vi "Testing Mode.vi"(8 "Filepath":path=path "D:/My Project/2019-2020/Magnetic Mareli UM/MM_UM/Project Setup/data/program seq/Program_280A.bin", 9 "FeedBack Channel":string[](array[string])=["fgdgfvcbc", "vnfhgjkn", "21354682"]) -> ()   [LabVIEW 2015]
uses:
  Control Button/Exit.ctl
  Control Button/Start.ctl
  Control Button/Home call.ctl
  Test  enqueue/AutoTest seq.ctl
  Control Button/Stop.ctl
  Control Button/Emergency.ctl
  Test  enqueue/Auot Test selection.ctl
  Galobal variable_TI.vi
  Project Setup/Globle Variable/GR_Servo.vi
panel:
  out "XY Graph":cluster{"X":dbl, "Y":dbl}[](graph)
  in  "Emergency":T1
  in  "Stop":T2
  out "Digital Output":bool[](array[boolean])
  out "D-enqueue":T3
  in  "Home Call":bool
  out "DI":bool[](array[boolean])
  in  "Home":T4
  out "Error Message":string
  out "Current Date & Time":timestamp
  out "Cycle Time(Sec)":i32
  in  "Start":T5
  in  "Cycle Start Bit":bool
  in  "vi reference":refnum<vi>
  in  "Reset Ct.":bool
  out "error out":errorcluster
  in  "Tbl Refnum":refnum<vi>
  in  "Table Control":string[][](table)
  out "User Name":string
  in  "Image Display":bool
  in  "Exit":T6
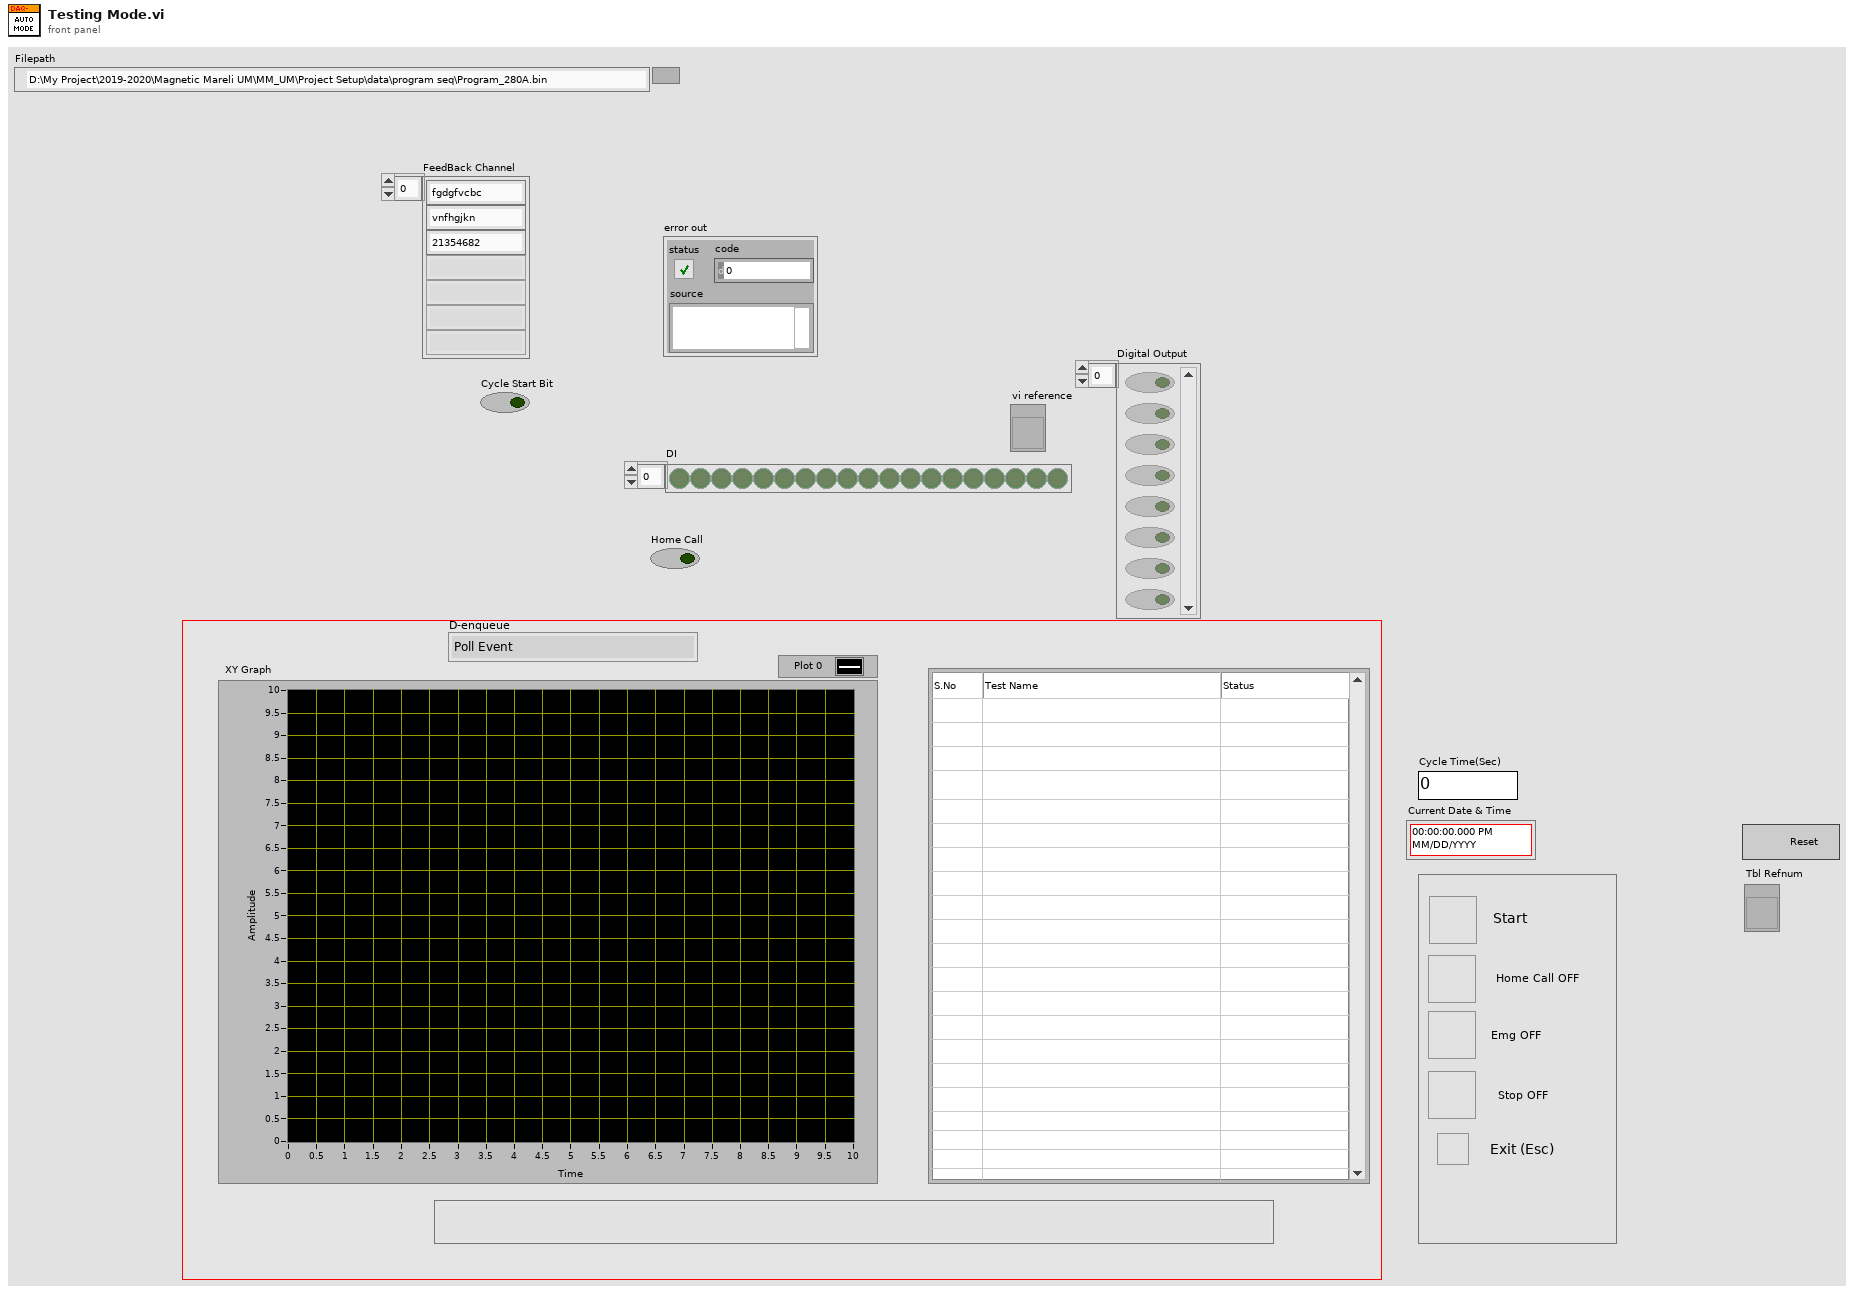
[diagram p1: front panel]
types:
  T1 = typedef "Emergency.ctl" = bool
  T2 = typedef "Stop.ctl" = bool
  T3 = typedef "AutoTest seq.ctl" = enum16{"Poll Event", "Initilization", "Cylender Home", "Read Barcode", "Slide Servo send Cammand", "Slide Servo Home Call", "LCD Press Servo send Cammand", "LCD Press. Servo Home Call", "Camera Co-ordinate_1", "Camera Co-ordinate_2", "Result Save", "Exit"}
  T4 = typedef "Home call.ctl" = bool
  T5 = typedef "Start.ctl" = bool
  T6 = typedef "Exit.ctl" = bool
  T7 = typedef "Auot Test selection.ctl" = enum16{"Init", "Enqueue ", "Enqueue N", "Enqueue in stack", "Enqueue in stack N", "Dequeue", "Dequeue N", "Flush", "Release Queue"}
  T8 = cluster{"Item Name":string, "Item Status":bool, "Steps":cluster{"Channel Type":string, "Channels":string, "Wait/Poll (ms)":u32, "Parameter":u8, "STM-Speed":i32, "STM-Degree":u32, "Direction":u8}[]}[]
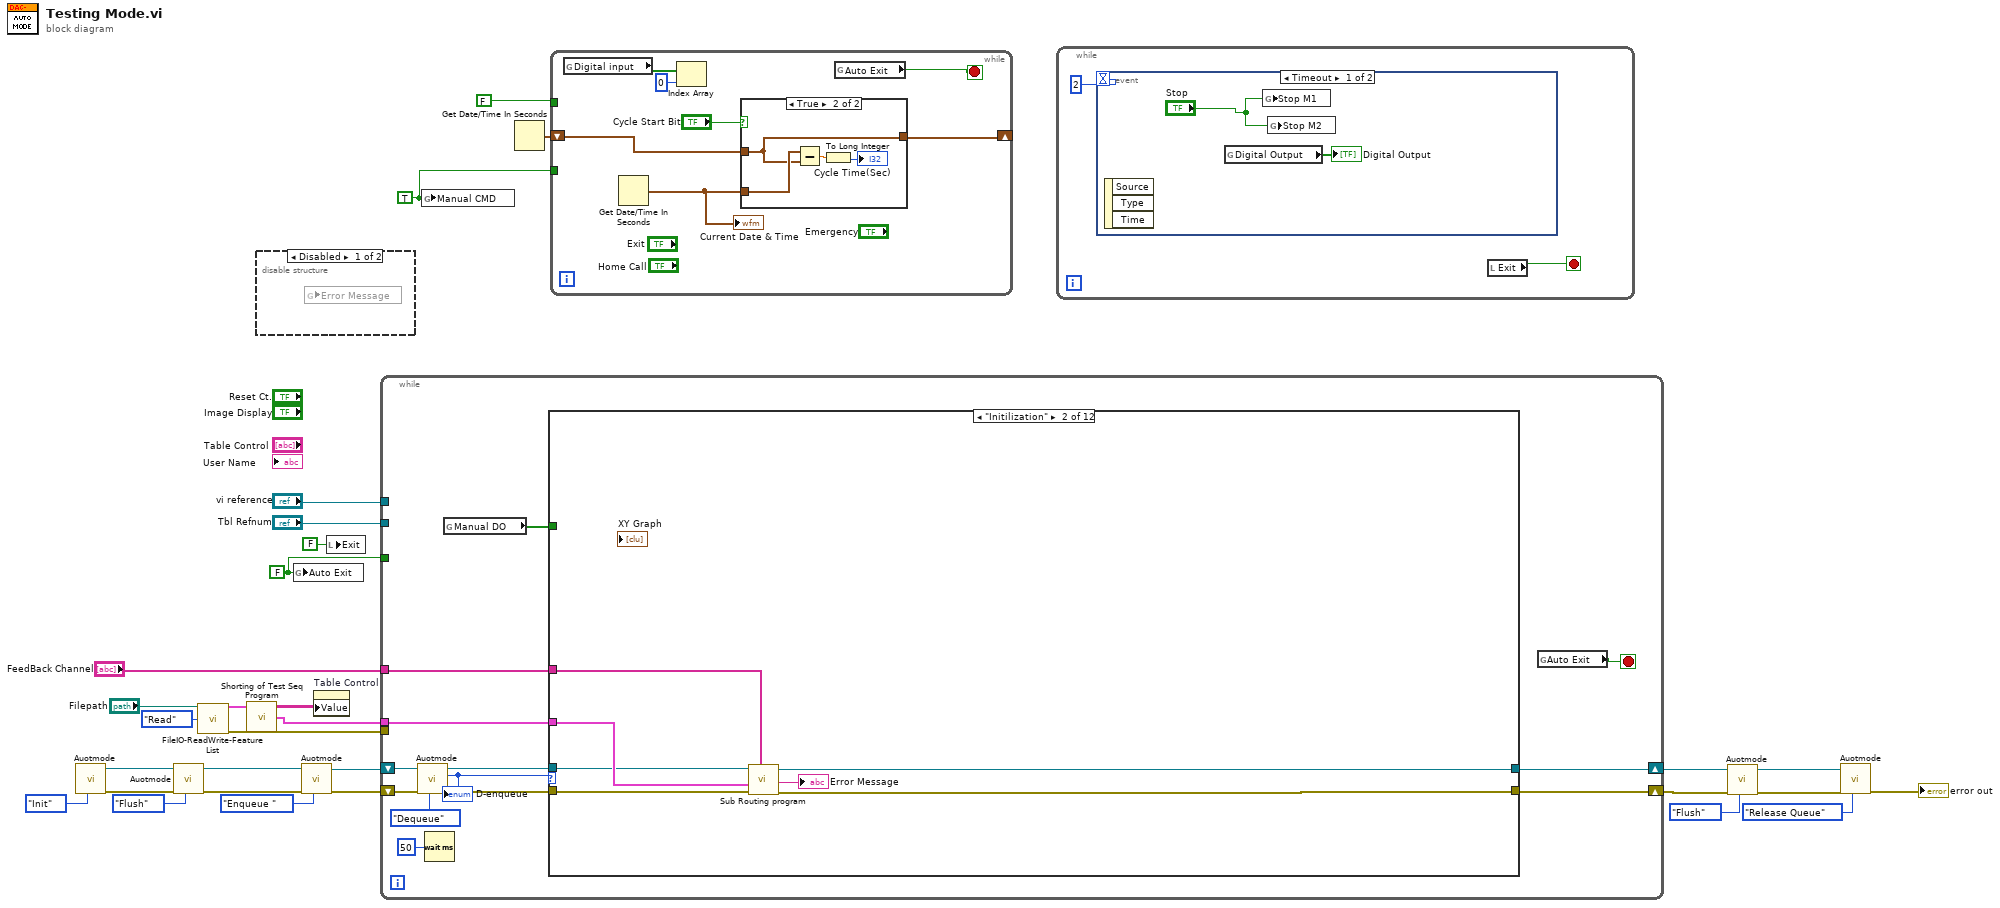
[diagram p0: block diagram]
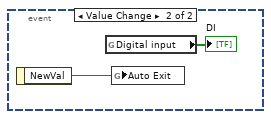
[diagram p3: hidden frame]
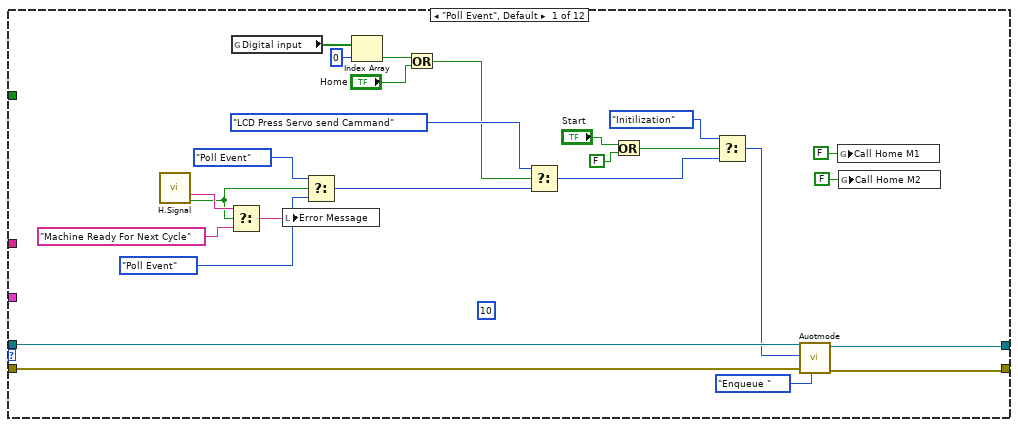
[diagram p5: hidden frame]
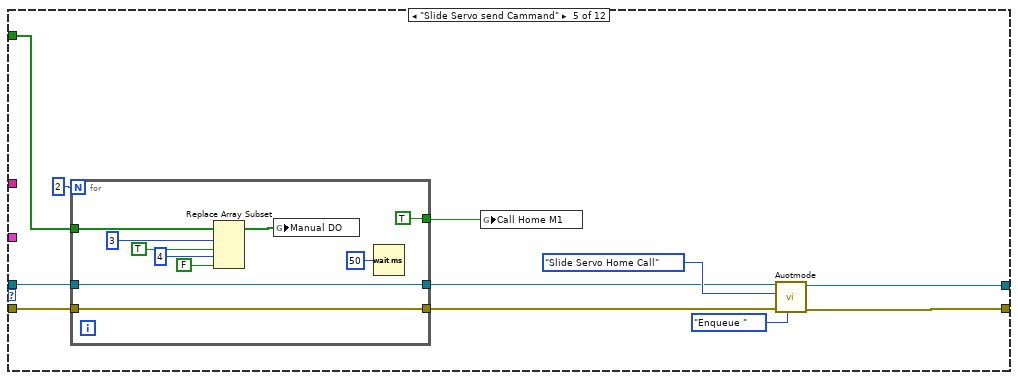
[diagram p8: hidden frame]
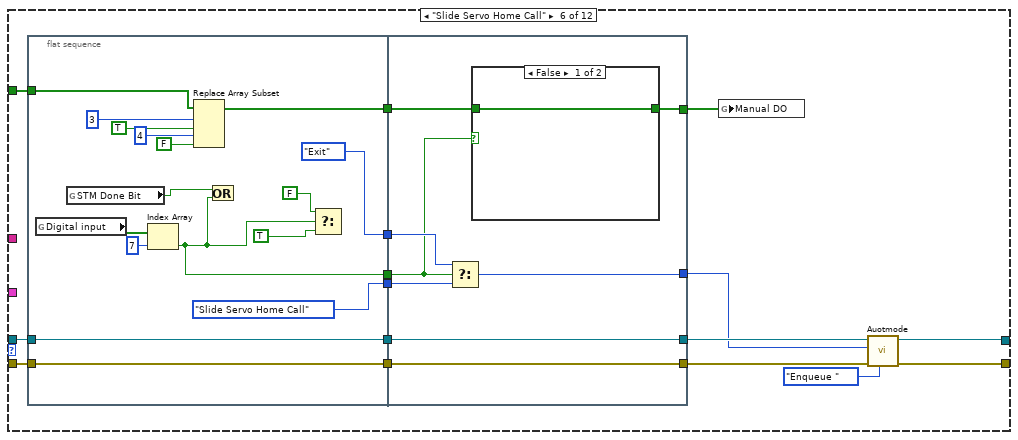
[diagram p9: hidden frame]
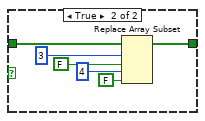
[diagram p10: hidden frame]
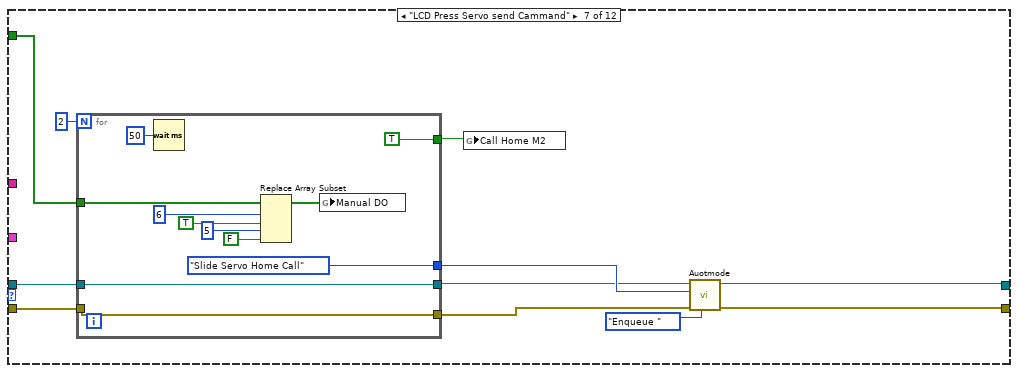
[diagram p11: hidden frame]
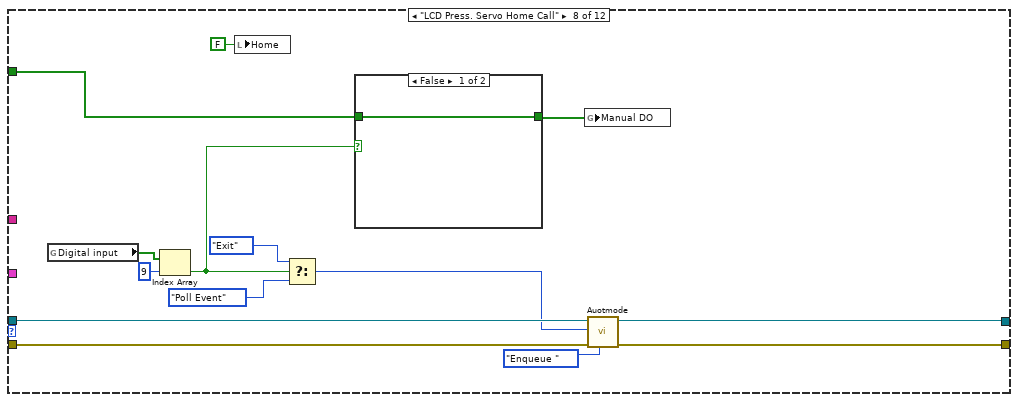
[diagram p12: hidden frame]
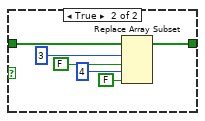
[diagram p13: hidden frame]
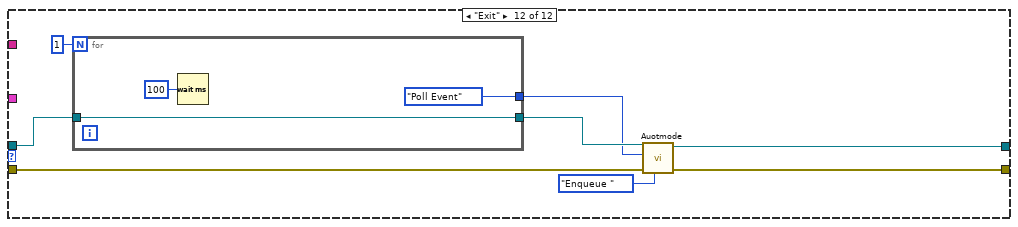
[diagram p17: hidden frame]
diagram:
  w2 = FALSE ("Auto Exit")
  w3 = TRUE ("Manual CMD")
  n1 = call "Auotmode.vi"("Enum Selection"=Auot_Test_selection."Init") -> ("error out"=w24:errorcluster, "queue Out"=w22:refnum<queue>)  [unwired: 7 in, 1 out]
  n2 = call "Auotmode.vi"("Enum Selection"=Auot_Test_selection."Flush", "Error In"=w24, "queue in"=w22) -> ("error out"=w23:errorcluster, "queue Out"=w21:refnum<queue>)  [unwired: 5 in, 1 out]
  n3 = call "FileIO-ReadWrite-FeatureList.vi"("Filepath"="Filepath", "Read/Write"=enum16{"Read", "Write"}."Read") -> ("Feature List (Out)"=w9:T8, "Error Out"=w11:errorcluster)  [unwired: 12 in]
  n4 = call "Shorting of Test Seq Program.vi"("Feature List (Out)"=w9) -> ("Feature Step Enable"=w7:T8, "Feature Name"=w8:string[][])  [unwired: 3 in]
  n5 = disable-structure shown="Disabled" {
    frame Disabled {
      n6 = global read "GR_Servo.vi" "Error Message"() -> ()  [unwired: 1 in]
    }
    frame Enabled {
    }
  }
  n7 = global write "Galobal variable_TI.vi" "Auto Exit"(w2) -> ()
  n8 = call "Auotmode.vi"("Enum Selection"=Auot_Test_selection."Enqueue ", "Error In"=w23, "queue in"=w21) -> ("error out"=w28:errorcluster, "queue Out"=w5:refnum<queue>)  [unwired: 5 in, 1 out]
  n9 = property on="Table Control" class="Tbl (strict)"("Value"=w8) -> ()  [unwired: 2 in, 2 out]
  n10 = local write "Exit"(T6 FALSE ("Exit")) -> ()
  n11 = while {
    tunnel: "vi reference" -> [_]
    tunnel: "Tbl Refnum" -> [_]
    tunnel: w7 -> [w36]
    tunnel: w11 -> [_]
    tunnel: "FeedBack Channel" -> [w37]
    shift-right: [w40] -> w15
    shift-left: w5 -> [w33]
    shift-right: [w32] -> w4
    shift-left: w28 -> [w42]
    tunnel: w2 -> [_]
    stop <- w35 stop-if-true
    n12 = call "Auotmode.vi"("Enum Selection"=Auot_Test_selection."Dequeue", "Error In"=w42, "queue in"=w33) -> ("error out"=w39:errorcluster, "D-enqueue"=w38:T3, "queue Out"=w41:refnum<queue>)  [unwired: 5 in]
    "D-enqueue" <- w38
    n13 = Wait (ms)(milliseconds to wait=u32 50) -> ()  [unwired: 1 out]
    n14 = global read "Galobal variable_TI.vi" "Manual DO"() -> (w31:bool[])
    n15 = case shown="\"Initilization\"" w38 {
      tunnel: w41 -> [w69 w70 w78 w80 w86 w114 w158 w180 w193 w195 w197 w201]
      tunnel: [w67 w73 w78 w80 w90 w115 w153 w179 w193 w195 w197 w202] -> w40
      tunnel: w39 -> [w68 w74 w77 w79 w83 w113 w157 w182 w192 w194 w196 w204]
      tunnel: [w66 w72 w77 w79 w89 w116 w152 w181 w192 w194 w196 w204] -> w32
      tunnel: w36 -> [_ w76 _ _ _ _ _ _ _ _ _ _]
      tunnel: w37 -> [_ w75 _ _ _ _ _ _ _ _ _ _]
      tunnel: w31 -> [_ _ _ _ w81 w103 w149 w172 _ _ _ _]
      frame "Poll Event", Default {
        (unwired) 10
        n16 = call "H.Signal.vi"() -> ("Error Message"=w50:string, "Bool_H Sig"=w47:bool)  [unwired: 11 in, 3 out]
        n17 = Select(t=w50, s=w47, f="Machine Ready For Next Cycle") -> (s? t:f=w48:string)
        n18 = global read "Galobal variable_TI.vi" "Digital input"() -> (w64:bool[])
        n19 = local write "Error Message"(w48) -> ()
        n20 = Select(t=AutoTest_seq."Poll Event" ("Enqueue"), s=w47, f=AutoTest_seq."Poll Event") -> (s? t:f=w45:T3)
        n21 = Index Array(array=w64, index=0) -> (element=w53:bool)
        n22 = Or(x=w53, y="Home") -> (x .or. y?=w51:T4)
        n23 = Select(t=AutoTest_seq."LCD Press Servo send Cammand" ("Enqueue"), s=w51, f=w45) -> (s? t:f=w56:T3)
        n24 = Or(x="Start", y=FALSE) -> (x .or. y?=w58:T5)
        n25 = Select(t=AutoTest_seq."Initilization" ("Enqueue"), s=w58, f=w56) -> (s? t:f=w55:T3)
        n26 = call "Auotmode.vi"("Enum Selection"=Auot_Test_selection."Enqueue ", "Error In"=w68, "Enqueue"=w55, "queue in"=w69) -> ("error out"=w66:errorcluster, "queue Out"=w67:refnum<queue>)  [unwired: 4 in, 1 out]
        n27 = global write "Galobal variable_TI.vi" "Call Home M1"(FALSE ("Call Home M1")) -> ()
        n28 = global write "Galobal variable_TI.vi" "Call Home M2"(FALSE ("Call Home M1")) -> ()
      }
      frame "Initilization" {
        n29 = call "Sub Routing program.vi"("FeedBack Channel"=w75, "error in (no error)"=w74, "Feature Step Enable"=w76, "queue Out in"=w70) -> ("error out"=w72:errorcluster, "Error Message"=→"Error Message":string, "Queue out"=w73:refnum<queue>)  [unwired: 5 in]
      }
      frame "Cylender Home" {
      }
      frame "Read Barcode" {
      }
      frame "Slide Servo send Cammand" {
        n30 = for {
          N: 2 -> [_]
          tunnel: [w100] -> w85
          tunnel: w86 -> [w100]
          tunnel: [TRUE ("Home Call")] -> w84
          tunnel: w83 -> [w94]
          tunnel: [w94] -> w82
          tunnel: w81 -> [w93]
          n31 = Replace Array Subset(array=w93, new element #1=TRUE ("new element/subarray"), index #1=3 ("index"), new element #2=FALSE ("new element/subarray"), index #2=4 ("index")) -> (w92:bool[])
          n32 = global write "Galobal variable_TI.vi" "Manual DO"(w92) -> ()
          n33 = Wait (ms)(milliseconds to wait=u32 50) -> ()  [unwired: 1 out]
        }
        n34 = global write "Galobal variable_TI.vi" "Call Home M1"(w84) -> ()
        n35 = call "Auotmode.vi"("Enum Selection"=Auot_Test_selection."Enqueue ", "Error In"=w82, "Enqueue"=AutoTest_seq."Slide Servo Home Call", "queue in"=w85) -> ("error out"=w89:errorcluster, "queue Out"=w90:refnum<queue>)  [unwired: 4 in, 1 out]
      }
      frame "Slide Servo Home Call" {
        n36 = flat-sequence {
          tunnel: w114 -> [w129]
          tunnel: w113 -> [w128]
          tunnel: [w129] -> w110
          tunnel: [w128] -> w109
          tunnel: [AutoTest_seq."Exit" ("Enqueue")] -> w108
          tunnel: [AutoTest_seq."Slide Servo Home Call" ("Enqueue")] -> w107
          tunnel: [w125] -> w106
          tunnel: [w119] -> w104
          tunnel: w103 -> [w118]
          tunnel: [w140] -> w111
          tunnel: [w141] -> w112
          tunnel: w110 -> [w141]
          tunnel: w109 -> [w140]
          tunnel: w108 -> [w139]
          tunnel: w107 -> [w138]
          tunnel: w106 -> [w136]
          tunnel: [w137] -> w105
          tunnel: w104 -> [w135]
          tunnel: [w134] -> w102
          frame #0 {
            n37 = global read "Galobal variable_TI.vi" "Digital input"() -> (w124:bool[])
            n38 = global read "Galobal variable_TI.vi" "STM Done Bit"() -> (w132:bool)
            n39 = Index Array(array=w124, index=7) -> (element=w125:bool)
            n40 = Replace Array Subset(array=w118, new element #1=TRUE ("new element/subarray"), index #1=3 ("index"), new element #2=FALSE ("new element/subarray"), index #2=4 ("index")) -> (w119:bool[])
            n41 = Or(x=w132, y=w125) -> ()  [unwired: 1 out]
            n42 = Select(t=FALSE, s=w125, f=TRUE) -> ()  [unwired: 1 out]
          }
          frame #1 {
            n43 = Select(t=w139, s=w136, f=w138) -> (s? t:f=w137:T3)
            n44 = case shown="False" w136 {
              tunnel: w135 -> [w142 w144]
              tunnel: [w142 w143] -> w134
              frame False {
              }
              frame True {
                n45 = Replace Array Subset(array=w144, new element #1=FALSE ("new element/subarray"), index #1=3 ("index"), new element #2=FALSE ("new element/subarray"), index #2=4 ("index")) -> (w143:bool[])
              }
            }
          }
        }
        n46 = global write "Galobal variable_TI.vi" "Manual DO"(w102) -> ()
        n47 = call "Auotmode.vi"("Enum Selection"=Auot_Test_selection."Enqueue ", "Error In"=w111, "Enqueue"=w105, "queue in"=w112) -> ("error out"=w116:errorcluster, "queue Out"=w115:refnum<queue>)  [unwired: 4 in, 1 out]
      }
      frame "LCD Press Servo send Cammand" {
        n48 = for {
          N: 2 -> [_]
          tunnel: [TRUE ("Home Call")] -> w150
          tunnel: [w168] -> w154
          tunnel: w158 -> [w168]
          tunnel: [w167] -> w151
          tunnel: w157 -> [w167]
          tunnel: [AutoTest_seq."Slide Servo Home Call" ("Enqueue")] -> w156
          tunnel: w149 -> [w161]
          n49 = Wait (ms)(milliseconds to wait=u32 50) -> ()  [unwired: 1 out]
          n50 = Replace Array Subset(array=w161, new element #1=TRUE ("new element/subarray"), index #1=6 ("index"), new element #2=FALSE ("new element/subarray"), index #2=5 ("index")) -> (w160:bool[])
          n51 = global write "Galobal variable_TI.vi" "Manual DO"(w160) -> ()
        }
        n52 = global write "Galobal variable_TI.vi" "Call Home M2"(w150) -> ()
        n53 = call "Auotmode.vi"("Enum Selection"=Auot_Test_selection."Enqueue ", "Error In"=w151, "Enqueue"=w156, "queue in"=w154) -> ("error out"=w152:errorcluster, "queue Out"=w153:refnum<queue>)  [unwired: 4 in, 1 out]
      }
      frame "LCD Press. Servo Home Call" {
        n54 = global read "Galobal variable_TI.vi" "Digital input"() -> (w177:bool[])
        n55 = Index Array(array=w177, index=9) -> (element=w173:bool)
        n56 = local write "Home"(FALSE ("Home")) -> ()
        n57 = Select(t=AutoTest_seq."Exit" ("Enqueue"), s=w173, f=AutoTest_seq."Poll Event") -> (s? t:f=w174:T3)
        n58 = case shown="False" w173 {
          tunnel: [w185 w187] -> w171
          tunnel: w172 -> [w185 w186]
          frame False {
          }
          frame True {
            n59 = Replace Array Subset(array=w186, new element #1=FALSE ("new element/subarray"), index #1=3 ("index"), new element #2=FALSE ("new element/subarray"), index #2=4 ("index")) -> (w187:bool[])
          }
        }
        n60 = global write "Galobal variable_TI.vi" "Manual DO"(w171) -> ()
        n61 = call "Auotmode.vi"("Enum Selection"=Auot_Test_selection."Enqueue ", "Error In"=w182, "Enqueue"=w174, "queue in"=w180) -> ("error out"=w181:errorcluster, "queue Out"=w179:refnum<queue>)  [unwired: 4 in, 1 out]
      }
      frame "Camera Co-ordinate_1" {
      }
      frame "Camera Co-ordinate_2" {
      }
      frame "Result Save" {
      }
      frame "Exit" {
        n62 = for {
          N: 1 -> [_]
          tunnel: w201 -> [w206]
          tunnel: [w206] -> w200
          tunnel: [AutoTest_seq."Poll Event" ("Enqueue")] -> w199
          n63 = Wait (ms)(milliseconds to wait=u32 100) -> ()  [unwired: 1 out]
        }
        n64 = call "Auotmode.vi"("Enum Selection"=Auot_Test_selection."Enqueue ", "Enqueue"=w199, "queue in"=w200) -> ("queue Out"=w202:refnum<queue>)  [unwired: 5 in, 2 out]
      }
    }
    n65 = global read "Galobal variable_TI.vi" "Auto Exit"() -> (w35:bool)
  }
  n66 = global write "Galobal variable_TI.vi" "Manual CMD"(w3) -> ()
  n67 = Get Date/Time In Seconds() -> (seconds since 1Jan1904=w14:timestamp)
  n68 = while {
    shift-right: [w212] -> _
    shift-left: w14 -> [w211]
    tunnel: w3 -> [_]
    tunnel: FALSE ("Servo Stop") -> [_]
    stop <- w209 stop-if-true
    n69 = global read "Galobal variable_TI.vi" "Digital input"() -> (w213:bool[])
    n70 = Get Date/Time In Seconds() -> (seconds since 1Jan1904=w208:timestamp)
    "Current Date & Time" <- w208
    n71 = Index Array(array=w213, index=0) -> ()  [unwired: 1 out]
    n72 = case shown="True" "Cycle Start Bit" {
      tunnel: w211 -> [_ w216]
      tunnel: w208 -> [w215 w217]
      tunnel: [w215 w216] -> w212
      frame False {
      }
      frame True {
        n73 = Subtract(x=w217, y=w216) -> (x-y=w219:dbl)
        n74 = To Long Integer(number=w219) -> (32bit integer=→"Cycle Time(Sec)":i32)
      }
    }
    n75 = global read "Galobal variable_TI.vi" "Auto Exit"() -> (w209:bool)
  }
  n76 = while {
    stop <- w221 stop-if-true
    n77 = event shown="[0] Timeout" {
      selector: _ -> [_ _]
      dyn-events: _ -> [_ _]
      timeout: 2 -> [_ _]
      event Timeout {
        n78 = event-data() -> ()  [unwired: 1 in, 3 out]
        n79 = global read "Galobal variable_TI.vi" "Digital Output"() -> (→"Digital Output":bool[])
        n80 = global write "Galobal variable_TI.vi" "Stop M1"("Stop") -> ()
        n81 = global write "Galobal variable_TI.vi" "Stop M2"("Stop") -> ()
      }
      event Value Change {
        n82 = event-data() -> ("NewVal"=w224:T6)  [unwired: 1 in]
        n83 = global read "Galobal variable_TI.vi" "Digital input"() -> (→"DI":bool[])
        n84 = global write "Galobal variable_TI.vi" "Auto Exit"(w224) -> ()
      }
    }
    n85 = local read "Exit"() -> (w221:T6)
  }
  n86 = call "Auotmode.vi"("Enum Selection"=Auot_Test_selection."Flush", "Error In"=w4, "queue in"=w15) -> ("error out"=w20:errorcluster, "queue Out"=w19:refnum<queue>)  [unwired: 5 in, 1 out]
  n87 = call "Auotmode.vi"("Enum Selection"=Auot_Test_selection."Release Queue", "Error In"=w20, "queue in"=w19) -> ("error out"=→"error out":errorcluster)  [unwired: 5 in, 2 out]
